vi "CODMn启动参数对话框.vi"() -> (1 "标样浓度输出":dbl, 2 "确认":bool, 3 "元素":cluster{"命令":string, "data":variant})   [LabVIEW 2016, in "斯坦道CODMn新电路板.lvlib"]
panel:
  in  "标样浓度":dbl
  in  "取消":bool
  in  "确定":bool
  in  "测量间隔":u16
  in  "模式设置":T1(ring)
  in  "量程切换":enum32{"H", "L", "AUTO"}(radio)=enum."AUTO"
  in  "站号":u16(ring)=21 items=["CODMn"=21]
  in  "控制命令":u16(ring)=1 items=["启动测量"=1, "标样核查"=2, "零点核查"=3, "跨度核查"=4, "空白测试"=5, "平行样测试"=6, "加标回收"=7, "空白校准"=8, "标样校准"=9, "初始化（清洗）"=10, "停止测试"=11, "仪器重启"=12, "校时"=13, "模式设置"=14, "测量间隔设置"=15, "调试"=22, "填充管路"=30, "清洗管路"=31, "清洗反应杯"=32]
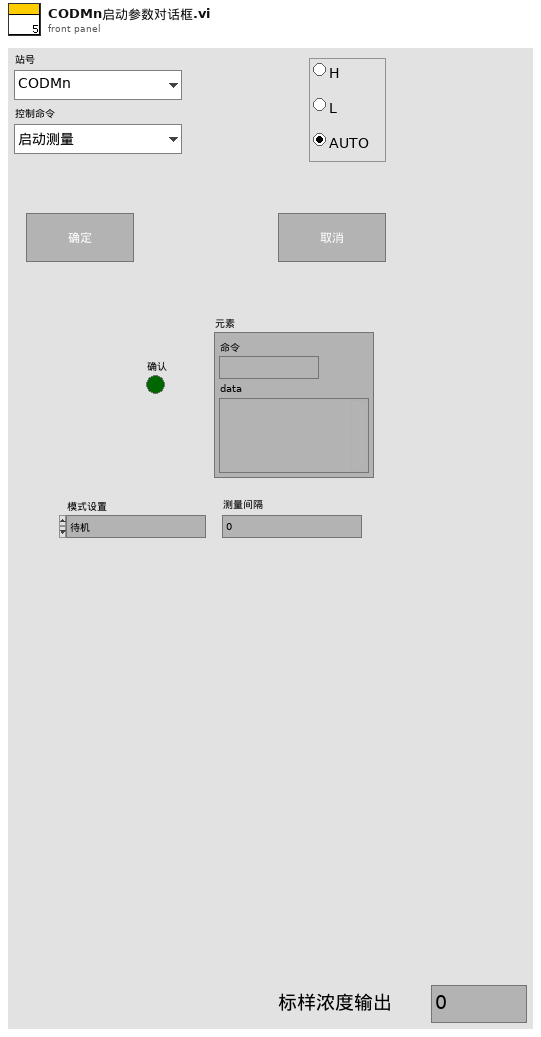
[diagram p1: front panel]
types:
  T1 = enum16{"待机", "连续模式", "周期模式", "定点模式", "受控模式", "手动模式"}
  T2 = cluster{"站号":u16, "量程切换":enum32{"H", "L", "AUTO"}, "控制命令":u16, "模式设置":enum16{"待机", "连续模式", "周期模式", "定点模式", "受控模式", "手动模式"}, "测量间隔":u16}
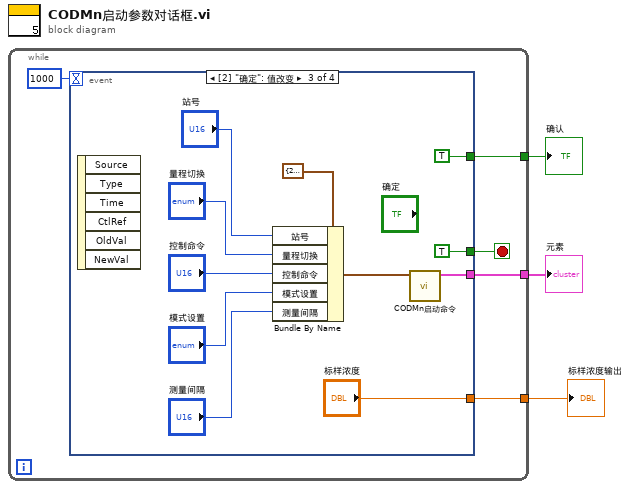
[diagram p0: block diagram]
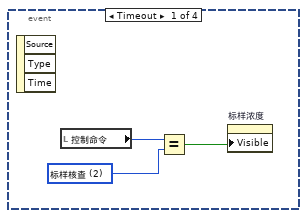
[diagram p2: hidden frame]
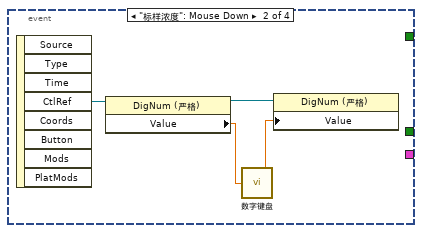
[diagram p3: hidden frame]
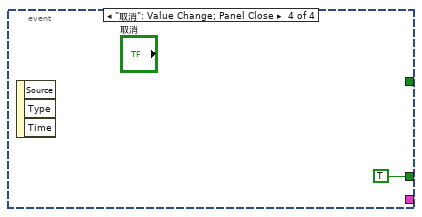
[diagram p4: hidden frame]
diagram:
  n1 = while {
    tunnel: [w6] -> w3
    tunnel: [w5] -> w2
    tunnel: [w4] -> w1
    stop <- w8 stop-if-true
    n2 = event shown="[2] \"确定\": 值改变" {
      selector: _ -> [_ _ _ _]
      dyn-events: _ -> [_ _ _ _]
      timeout: 1000 -> [_ _ _ _]
      tunnel: [_ _ TRUE TRUE] -> w8
      tunnel: [_ _ TRUE _] -> w6
      tunnel: [_ _ w24 _] -> w5
      tunnel: [_ _ "标样浓度" _] -> w4
      event Timeout {
        w10 = u16 2 items=["启动测量"=1, "标样核查"=2, "零点核查"=3, "跨度核查"=4, "空白测试"=5, "平行样测试"=6, "加标回收"=7, "空白校准"=8, "标样校准"=9, "初始化（清洗）"=10, "停止测试"=11, "仪器重启"=12, "校时"=13, "模式设置"=14, "测量间隔设置"=15, "调试"=22, "填充管路"=30, "清洗管路"=31, "清洗反应杯"=32] ("控制命令")
        n3 = event-data() -> ()  [unwired: 1 in, 3 out]
        n4 = local read "控制命令"() -> (w11:u16)
        n5 = Equal?(x=w11, y=w10) -> (x = y?=w9:bool)
        n6 = property on="标样浓度" class="DigNum (严格)"("Visible"=w9) -> ()  [unwired: 2 in, 2 out]
      }
      event "标样浓度": Mouse Down {
        n7 = event-data() -> ("CtlRef"=w15:refnum<vi>)  [unwired: 1 in, 7 out]
        n8 = property class="DigNum (严格)"(reference=w15) -> (reference out=w14:refnum<vi>, "Value"=w13:dbl)  [unwired: 1 in, 1 out]
        n9 = call "数字键盘.vi"("OldNumber"=w13) -> ("NewNumber"=w12:dbl)
        n10 = property class="DigNum (严格)"(reference=w14, "Value"=w12) -> ()  [unwired: 1 in, 2 out]
      }
      event "确定": Value Change {
        n11 = event-data() -> ()  [unwired: 1 in, 6 out]
        n12 = Bundle By Name(cluster=T2 {"站号"=21, "量程切换"=enum."AUTO", "控制命令"=1, "模式设置"=enum."待机", "测量间隔"=0} ("参数"), "站号"="站号", "量程切换"="量程切换", "控制命令"="控制命令", "模式设置"="模式设置", "测量间隔"="测量间隔") -> (w22:T2)
        n13 = call "CODMn启动命令.vi"("参数"=w22) -> ("启动命令"=w24:cluster{"命令":string, "data":variant})  [unwired: 10 in]
      }
      event "取消": Value Change; Panel Close {
        n14 = event-data() -> ()  [unwired: 1 in, 3 out]
      }
    }
  }
  "元素" <- w2
  "确认" <- w3
  "标样浓度输出" <- w1
